vi "test.vi"(11 "Data In":i32) -> (3 "Data Out":i32)   [LabVIEW 2016]
doc: "Assert Component\nAssert Name: test\nData Type: I32\nDeveloped by UKHornP\nEvaluation String: X = 12\nDescription: hello blah blah blah"
uses:
  Core/Assert API Components/Failure Actions.ctl
  Core/Assert API Components/VI References.ctl
  Core/Assert API Components/Assert API Components.lvlib
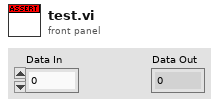
[diagram p1: front panel]
types:
  T1 = typedef "Assert API Components.lvlib/VI References.ctl" = cluster{"Calling VI Ref":refnum<vi>, "Assert VI Ref":refnum<vi>}
  T2 = typedef "Assert API Components.lvlib/Failure Actions.ctl" = enum16{"None", "Log To File", "Pause Execution", "Abort Execution"}
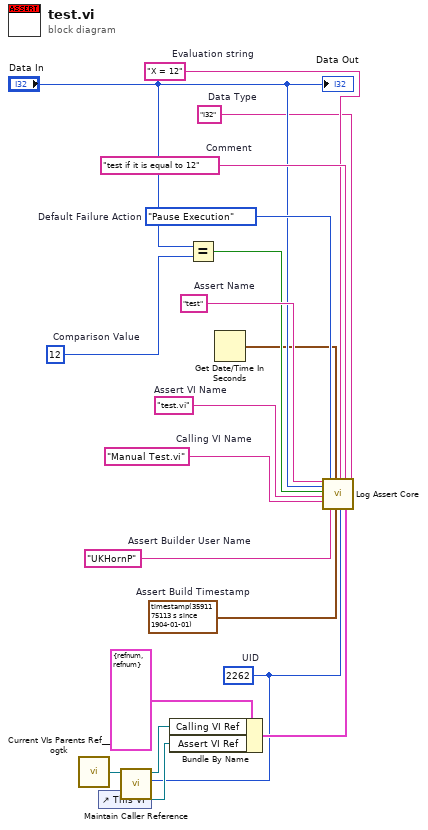
[diagram p0: block diagram]
diagram:
  w1 = 2262  # UID
  w4 = "test.vi"  # Assert VI Name
  w5 = "Manual Test.vi"  # Calling VI Name
  w6 = timestamp(3591175113.2770233 s since 1904-01-01)  # Assert Build Timestamp
  w7 = "UKHornP"  # Assert Builder User Name
  w8 = "I32"  # Data Type
  w16 = "test if it is equal to 12"  # Comment
  w13 = "X = 12"  # Evaluation string
  w18 = Failure_Actions."Pause Execution"  # Default Failure Action
  w19 = "test"  # Assert Name
  w17 = 12  # Comparison Value
  n1 = call <userlib>:"Current VIs Parents Ref__ogtk.vi"() -> ("Calling VI's Reference"=w11:refnum<vi>)  [unwired: 2 in]
  n2 = control-ref of="This VI"() -> (w10:refnum<vi>)
  n3 = call "Maintain Caller Reference.vi"("UID"=w1, "VI in"=w11) -> ("VI out"=w3:refnum<vi>)  [unwired: 9 in]
  n4 = Bundle By Name(cluster=T1 {"Calling VI Ref"=refnum, "Assert VI Ref"=refnum} ("VI References"), "Calling VI Ref"=w3, "Assert VI Ref"=w10) -> (w9:T1)
  n5 = Equal?(x="Data In", y=w17) -> (x = y?=w14:bool)
  n6 = Get Date/Time In Seconds() -> (seconds since 1Jan1904=w2:timestamp)
  n7 = call "Log Assert Core.vi"("Assert Name"=w19, "Data Value"="Data In", "Status"=w14, "Assert VI Name"=w4, "Calling VI Name"=w5, "Failure Action"=w18, "Assert Builder User Name"=w7, "Last Update"=w2, "Assert Build Timestamp"=w6, "Evaluation String"=w13, "Assert VI UID"=w1, "Comment"=w16, "VI References"=w9, "Data Type"=w8) -> ()  [unwired: 6 in]
  "Data Out" <- "Data In"
